vi "GetdBBoost.vi"(8 "错误输入（无错误）":errorcluster) -> (0 "错误输出":errorcluster)   [LabVIEW 2014]
uses:
  X86Dll/ZXUTConfigMgr.dll
panel:
  out "返回值":i32
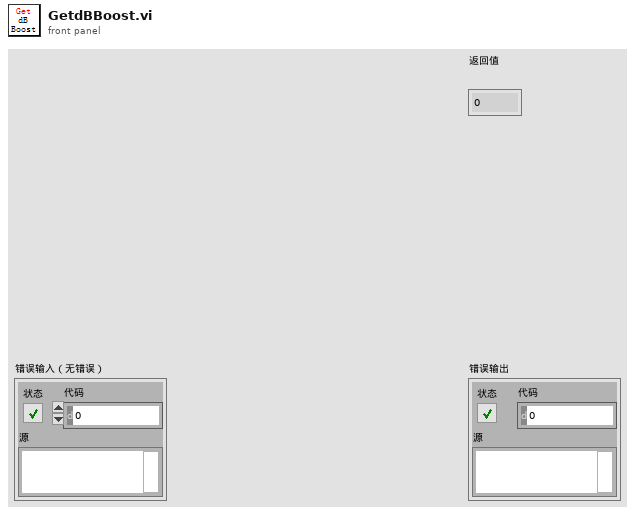
[diagram p1: front panel]
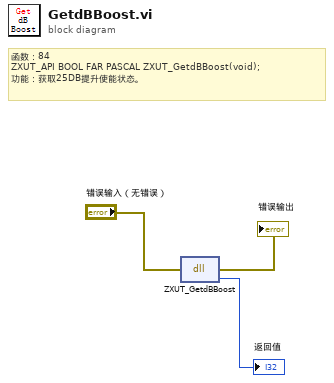
[diagram p0: block diagram]
diagram:
  # "函数：84\nZXUT_API BOOL\tFAR PASCAL ZXUT_GetdBBoost(void);\n功能：获取25DB提升使能状态。"
  n1 = dll-call lib="D:/Software/Utrasonic on-line monitoring/X86Dll/ZXUTConfigMgr.dll" fn="ZXUT_GetdBBoost"(error in="错误输入（无错误）") -> (error out=→"错误输出":errorcluster, "返回值"=→"返回值":i32)  [unwired: 2 in, 1 out]
